vi "approach 1.vi"() -> ()   [LabVIEW 2024]
uses:
  <vilib>/measure/mamon.llb/Waveform Peak Detection for 1 Chan.vi
  <vilib>/measure/NI_MAPro.lvlib
panel:
  in  "stop(F)":bool
  out "dt2":dbl
  out "subtraction":dbl
  out "Waveform Graph":dynamicdata(graph)
  out "x*y":dbl
  out "bpm":dbl
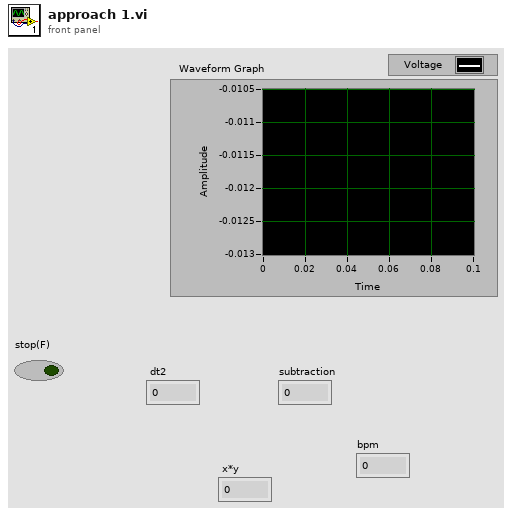
[diagram p1: front panel]
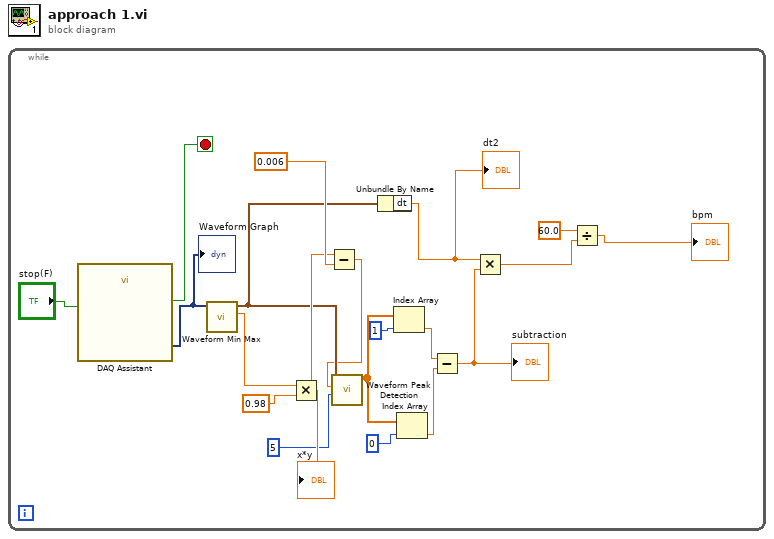
[diagram p0: block diagram]
diagram:
  n1 = while {
    stop <- w1 stop-if-true
    n2 = call "DAQ Assistant"("stop (F)"="stop(F)") -> ("data"=w3:dynamicdata, "stopped"=w1:bool)  [unwired: 15 in, 2 out]
    "Waveform Graph" <- w3
    n3 = call <vilib>:"Waveform Min Max.vi"("waveform in"=w3) -> ("Y max"=w13:dbl, "waveform out"=w9:waveform(dbl))  [unwired: 5 in, 4 out]
    n4 = Multiply(x=w13, y=0.98) -> (x*y=w10:dbl)
    "x*y" <- w10
    n5 = Subtract(x=w10, y=0.006) -> (x-y=w7:dbl)
    n6 = call-poly <vilib>:"Waveform Peak Detection.vi"("width"=5, "threshold"=w7, "Signal In"=w9) -> ("Locations"=w8:dbl[])  [unwired: 4 in, 4 out]
    n7 = Unbundle By Name(w9) -> ("dt"=w17:dbl)
    "dt2" <- w17
    n8 = Index Array(array=w8, index=1) -> (element=w6:dbl)
    n9 = Index Array(array=w8, index=0) -> (element=w5:dbl)
    n10 = Subtract(x=w6, y=w5) -> (x-y=w16:dbl)
    "subtraction" <- w16
    n11 = Multiply(x=w17, y=w16) -> (x*y=w18:dbl)
    n12 = Divide(x=60.0, y=w18) -> (x/y=→"bpm":dbl)
  }
